vi "Write Message Priority.vi"(8 "error in (no error)":errorcluster, 10 "Priority":u16=1, 11 "Sequencer Msg in":refnum<class "Sequencer Msg.lvclass">) -> (0 "error out":errorcluster, 3 "Sequencer Msg out":refnum<class "Sequencer Msg.lvclass">)   [LabVIEW 2020, in "Sequencer.lvlib" / "Sequencer Msg.lvclass"]
doc: "Write the Message Priority to the Sequencer Msg"
uses:
  Sequencer Msg.lvclass
  Sequencer Msg.lvclass/Sequencer Msg.ctl
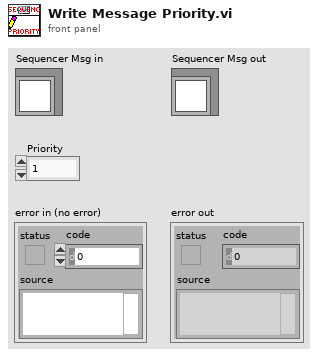
[diagram p1: front panel]
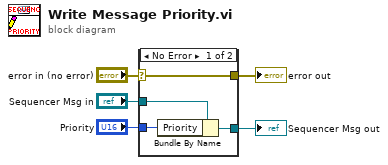
[diagram p0: block diagram]
diagram:
  n1 = case shown="No Error" "error in (no error)" {
    selector: "error in (no error)" -> [w9 w10]
    tunnel: [w9 w10] -> w4
    tunnel: [w7 w11] -> w2
    tunnel: "Sequencer Msg in" -> [w8 w11]
    tunnel: "Priority" -> [w6 _]
    frame No Error {
      n2 = Bundle By Name(cluster=w8, "Priority"=w6) -> (w7:refnum<class "Sequencer Msg.lvclass">)
    }
    frame Error {
    }
  }
  "error out" <- w4
  "Sequencer Msg out" <- w2
